vi "Destroy Subpanel.vi"(8 "error in (no error)":errorcluster, 11 "CIF_UI in":refnum<class "CIF_UI.lvclass">) -> (0 "error out":errorcluster, 3 "CIF_UI out":refnum<class "CIF_UI.lvclass">)   [LabVIEW 2021, in "CIF_UI.lvclass"]
uses:
  CIF_UI.lvclass
  CIF_UI.lvclass/CIF_UI.ctl
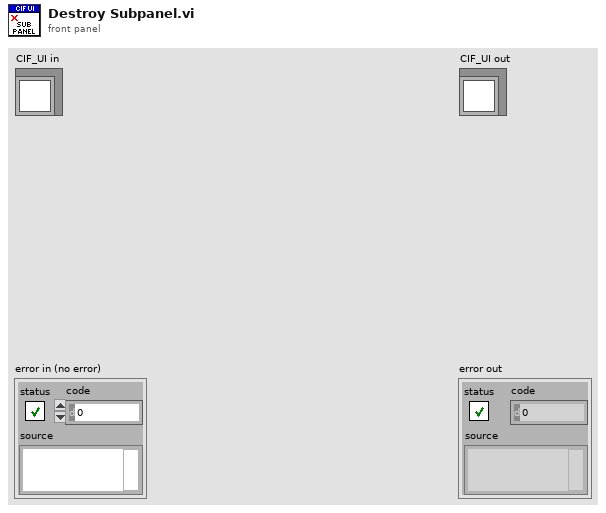
[diagram p1: front panel]
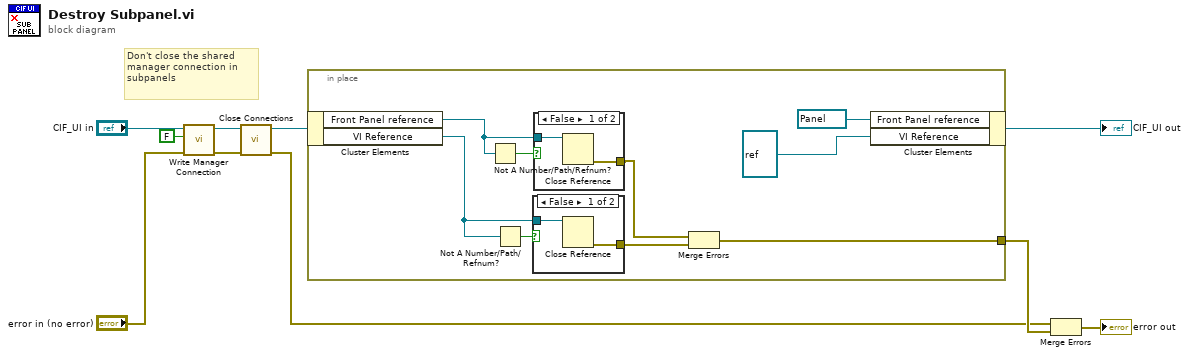
[diagram p0: block diagram]
diagram:
  # "Don't close the shared manager connection in subpanels"
  n1 = call "Write Manager Connection.vi"("error in (no error)"="error in (no error)", "Manager Connection"=FALSE, "CIF_UI in"="CIF_UI in") -> ("error out"=w3:errorcluster, "CIF_UI out"=w4:refnum<class "CIF_UI.lvclass">)  [unwired: 7 in]
  n2 = call "Close Connections.vi"("error in (no error)"=w3, "CIF_UI in"=w4) -> ("error out"=w7:errorcluster, "CIF_UI out"=w6:refnum<class "CIF_UI.lvclass">)  [unwired: 8 in]
  n3 = in-place {
    in-place-border: [w11] -> w9
    n4 = in-place-cluster #1(w6) -> ("Front Panel reference"=w16:refnum<vi>, "VI Reference"=w18:refnum<vi>)
    n5 = Not A Number/Path/Refnum?(number/path/refnum=w16) -> (NaN/Path/Refnum?=w17:bool)
    n6 = Not A Number/Path/Refnum?(number/path/refnum=w18) -> (NaN/Path/Refnum?=w19:bool)
    n7 = case shown="False" w19 {
      tunnel: w18 -> [w23 _]
      tunnel: [w22 _] -> w13
      frame False {
        n8 = Close Reference(reference=w23) -> (error out=w22:errorcluster)  [unwired: 1 in]
      }
      frame True {
      }
    }
    n9 = case shown="False" w17 {
      tunnel: w16 -> [w21 _]
      tunnel: [w20 _] -> w12
      frame False {
        n10 = Close Reference(reference=w21) -> (error out=w20:errorcluster)  [unwired: 1 in]
      }
      frame True {
      }
    }
    n11 = Merge Errors(w12, w13) -> (w11:errorcluster)
    n12 = in-place-cluster #1("Front Panel reference"=refnum<vi> refnum, "VI Reference"=refnum<vi> refnum) -> (→"CIF_UI out":refnum<class "CIF_UI.lvclass">)
  }
  n13 = Merge Errors(w7, w9) -> (→"error out":errorcluster)
